vi "Ridders Zero Finder.vi"   [LabVIEW 2020, in "NI_Gmath.lvlib"]
doc: "Determines a zero of a 1D function in a given interval. The function has to be continuous and has to have different signs at the end points of the interval. You must manually select the polymorphic instance to use."
uses:
  NI_Gmath.lvlib
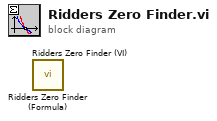
[diagram p0: block diagram]
diagram:
  n1 = call "Ridders Zero Finder (Formula).vi"() -> ()  [unwired: 8 in, 4 out]
  n2 = call "Ridders Zero Finder (VI).vi"() -> ()  [unwired: 8 in, 4 out]
